vi "DtCreateCtrRateChan.vi"(1 "Requested\nFrequency (Hz)":dbl=1000.0, 2 "Duty Cycle":dbl(slide)=50.0 scale=0.0..100.0, 5 "Board Name":string, 7 "Counter Num":u32, 9 "Gate Type":i32(ring)=2 items=["LowLevel", "HighLevel", "None"], 11 "error in (no error)":errorcluster) -> (4 "Task out":i32, 6 "Actual\nFrequency (Hz)":dbl, 15 "error out":errorcluster)   [LabVIEW 2022 SP3]
doc: "Creates one or more virtual counter/timer channels that generate output pulses continuously at a specified frequency (in Hz) when the counter/timer is enabled (determined by the counter/timer's gate input signal)."
uses:
  DtLvLink.lvlib
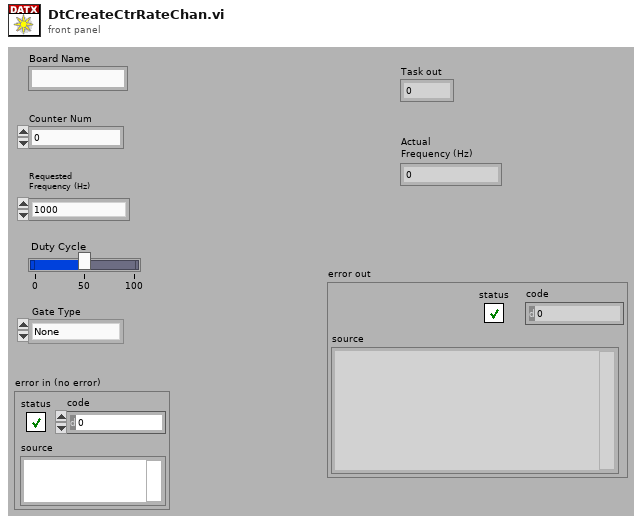
[diagram p1: front panel]
types:
  T1 = enum32{"AnalogInput", "AnalogOutput", "DigitalInput", "DigitalOutput", "Quadrature", "CounterTimer"}
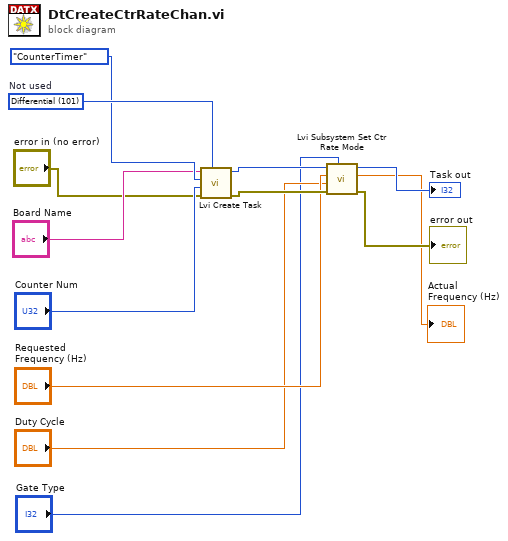
[diagram p0: block diagram]
diagram:
  w13 = 101 items=["SingleEnded"=100, "Differential"=101]  # Not used
  n1 = call "Lvi Create Task.vi"("SEorDiff"=w13, "error in (no error)"="error in (no error)", "SubSysIndex"="Counter Num", "ChanType"=T1."CounterTimer", "BoardName"="Board Name") -> ("error out"=w8:errorcluster, "TaskRef"=w7:i32)  [unwired: 4 in, 1 out]
  n2 = call "Lvi Subsystem Set Ctr Rate Mode.vi"("GateLevel"="Gate Type", "error in (no error)"=w8, "DutyCycle"="Duty Cycle", "Frequency"="Requested\nFrequency (Hz)", "TaskRef"=w7) -> ("error out"=→"error out":errorcluster, "ActualFrequency"=→"Actual\nFrequency (Hz)":dbl, "TaskRef out"=→"Task out":i32)  [unwired: 3 in, 1 out]
